vi "get VIA.vi"(11 "IO in":refnum<class "IO.lvclass">) -> (3 "Memory":refnum<class "Memory.lvclass">)   [LabVIEW 2021, in "IO.lvclass"]
uses:
  IO.lvclass
  Memory/Memory.lvclass
  IO.lvclass/IO.ctl
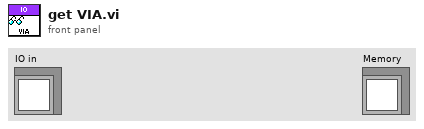
[diagram p1: front panel]
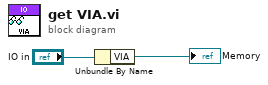
[diagram p0: block diagram]
diagram:
  n1 = Unbundle By Name("IO in") -> ("VIA"=→"Memory":refnum<class "Memory.lvclass">)
